vi "attribute_read_int32.vi"(5 "Repeated Capability":string, 7 "Attribute":T1={"Identifier"="", "Descriptive name"="", "Data Type"=enum."Integer 32", "Command"="", "Access"=2, "Range Table"="", "Read Callback"="", "Write Callback"="", "Range Callback"="", "Check Callback"="", "Rngtable Callback"="", "Coerce Callback"="", "Supported Models"="", "Instrument Options"="", "Repeated Capabilities"="", "Check Status Callback"="", "Index"=0, "Flag: OPC Wait"=FALSE, "Flag: Dont check status"=FALSE, "Flag: Cache Only"=FALSE} {"Access" items=["Read Only", "Write Only", "Read/Write"]}, 8 "error in":errorcluster, 11 "VISA resource name":refnum<visa-resource-name>) -> (0 "error out":errorcluster, 2 "I32 out":i32, 3 "VISA resource name out":refnum<visa-resource-name>)   [LabVIEW 2014, in "rszvl_rsidr_core.lvlib"]
uses:
  rszvl_rsidr_core.lvlib
  type_Attribute.ctl
  type_Attribute_Data_Type.ctl
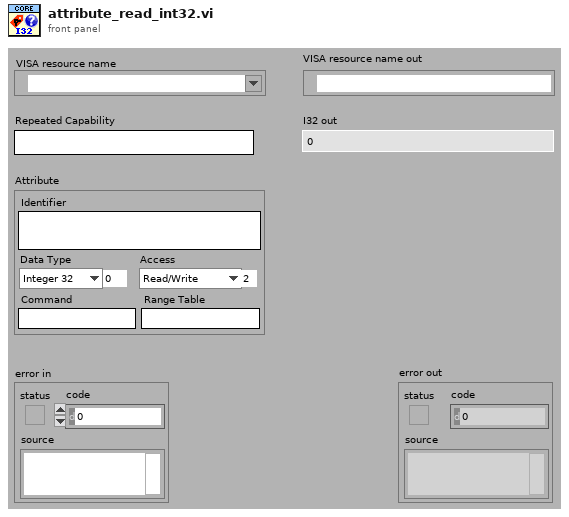
[diagram p1: front panel]
types:
  T1 = typedef "rszvl_rsidr_core.lvlib/type_Attribute.ctl" = cluster{"Identifier":string, "Descriptive name":string, "Data Type":T2, "Command":string, "Access":u16, "Range Table":string, "Read Callback":string, "Write Callback":string, "Range Callback":string, "Check Callback":string, "Rngtable Callback":string, "Coerce Callback":string, "Supported Models":string, "Instrument Options":string, "Repeated Capabilities":string, "Check Status Callback":string, "Index":i32, "Flag: OPC Wait":bool, "Flag: Dont check status":bool, "Flag: Cache Only":bool}
  T2 = typedef "rszvl_rsidr_core.lvlib/type_Attribute_Data_Type.ctl" = enum16{"Integer 32", "Double", "String", "Boolean", "None", "Integer 64"}
  T3 = typedef "rszvl_rsidr_core.lvlib/type_Session_Data.ctl" = cluster{"Instr type":string, "Instr type for err. msg.":string, "Installed Options":string[], "OPC Timeout":i32, "Query Instrument Status":bool, "Check Range":bool, "Check Options":bool, "Add LF to Write":bool, "Simulate":bool, "Logging":bool, "Logging params":variant, "Interface Type":enum16{"Unknown", "GPIB", "VXI", "GPIB_VXI", "ASRL", "PXI", "TCPIP", "USB", "SOCKET"}, "Fast Sweep":i32, "AdditionalFlags":i32, "WaitBeforeWrite":i32, "WaitBeforeRead":i32, "BinDataChunkSize":i64}
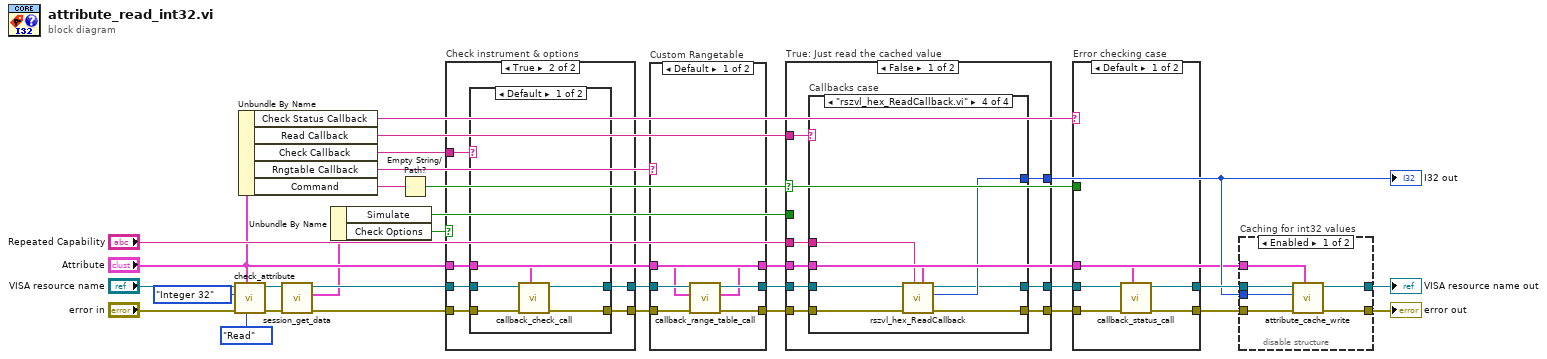
[diagram p0: block diagram]
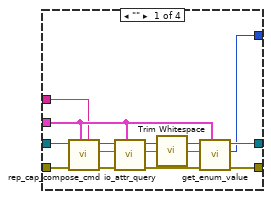
[diagram p2: hidden frame]
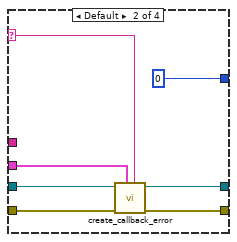
[diagram p3: hidden frame]
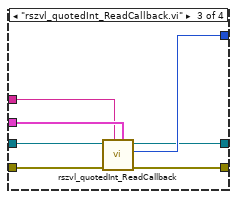
[diagram p4: hidden frame]
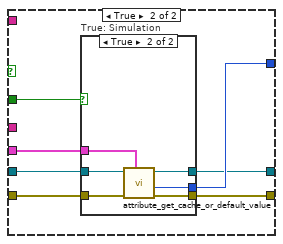
[diagram p5: hidden frame]
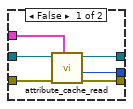
[diagram p6: hidden frame]
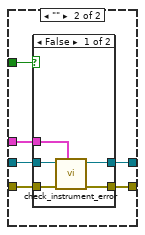
[diagram p8: hidden frame]
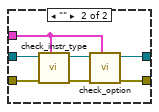
[diagram p11: hidden frame]
diagram:
  n1 = call "check_attribute.vi"("Access"=enum16{"Read", "Write"}."Read", "Attribute"="Attribute", "error in"="error in", "Data Type"=type_Attribute_Data_Type."Integer 32", "VISA resource name"="VISA resource name") -> ("error out"=w16:errorcluster, "VISA resource name out"=w17:refnum<visa-resource-name>)  [unwired: 5 in]
  n2 = Unbundle By Name("Attribute") -> ("Check Status Callback"=w18:string, "Read Callback"=w19:string, "Check Callback"=w7:string, "Rngtable Callback"=w8:string, "Command"=w3:string)
  n3 = call "session_get_data.vi"("error in"=w16, "VISA resource name"=w17) -> ("error out"=w15:errorcluster, "Session User Data out"=w2:T3, "VISA resource name out"=w14:refnum<visa-resource-name>)  [unwired: 7 in]
  n4 = Unbundle By Name(w2) -> ("Simulate"=w1:bool, "Check Options"=w13:bool)
  n5 = Empty String/Path?(string/path=w3) -> (empty?=w28:bool)
  n6 = case "Check instrument & options" shown="True" w13 {
    tunnel: [w33 w39] -> w12
    tunnel: [w32 w38] -> w11
    tunnel: w7 -> [_ w37]
    tunnel: w15 -> [w32 w36]
    tunnel: w14 -> [w33 w35]
    tunnel: "Attribute" -> [_ w34]
    frame False {
    }
    frame True {
      n7 = case shown="Default" w37 {
        tunnel: [w43 w49] -> w39
        tunnel: [w41 w48] -> w38
        tunnel: w36 -> [w42 w47]
        tunnel: w35 -> [w44 w46]
        tunnel: w34 -> [w40 w45]
        frame Default {
          n8 = call "callback_check_call.vi"("Attribute"=w40, "error in"=w42, "VISA resource name"=w44) -> ("error out"=w41:errorcluster, "VISA resource name out"=w43:refnum<visa-resource-name>)  [unwired: 7 in]
        }
        frame "" {
          n9 = call "check_instr_type.vi"("Attribute"=w45, "error in"=w47, "VISA resource name"=w46) -> ("error out"=w51:errorcluster, "VISA resource name out"=w50:refnum<visa-resource-name>)  [unwired: 6 in, 1 out]
          n10 = call "check_option.vi"("Attribute"=w45, "error in"=w51, "VISA resource name"=w50) -> ("error out"=w48:errorcluster, "VISA resource name out"=w49:refnum<visa-resource-name>)  [unwired: 7 in]
        }
      }
    }
  }
  n11 = case "Custom Rangetable" shown="Default" w8 {
    tunnel: w12 -> [w57 w60]
    tunnel: w11 -> [w54 w59]
    tunnel: [w56 w60] -> w10
    tunnel: [w55 w59] -> w9
    tunnel: "Attribute" -> [w53 w58]
    tunnel: [w52 w58] -> w6
    frame Default {
      n12 = call "callback_range_table_call.vi"("error in"=w54, "Attribute in"=w53, "VISA resource name"=w57) -> ("error out"=w55:errorcluster, "Attribute out"=w52:T1, "VISA resource name out"=w56:refnum<visa-resource-name>)  [unwired: 6 in]
    }
    frame "" {
    }
  }
  n13 = case "True: Just read the cached value" shown="False" w28 {
    tunnel: "Repeated Capability" -> [w68 _]
    tunnel: [w67 w106] -> w21
    tunnel: [w66 w105] -> w20
    tunnel: [w65 w107] -> w23
    tunnel: w19 -> [w64 _]
    tunnel: w10 -> [w63 w109]
    tunnel: w9 -> [w62 w110]
    tunnel: w6 -> [w61 w108]
    tunnel: w1 -> [_ w104]
    frame False {
      n14 = case "Callbacks case" shown="\"rszvl_hex_ReadCallback.vi\"" w64 {
        selector: w64 -> [_ w84 _ _]
        tunnel: w63 -> [w82 w88 w95 w102]
        tunnel: w62 -> [w81 w89 w96 w103]
        tunnel: w68 -> [w74 _ w93 w100]
        tunnel: [w80 w86 w90 w97] -> w66
        tunnel: [w79 w87 w91 w98] -> w67
        tunnel: [w69 0 ("Attribute Value I32") w92 w99] -> w65
        tunnel: w61 -> [w75 w85 w94 w101]
        frame "" {
          n15 = call "rep_cap_compose_cmd.vi"("Repeated Capability"=w74, "Attribute"=w75, "error in"=w81, "VISA resource name"=w82) -> ("error out"=w78:errorcluster, "Command out"=w77:string, "VISA resource name out"=w76:refnum<visa-resource-name>)  [unwired: 5 in]
          n16 = call "io_attr_query.vi"("Attribute"=w75, "error in"=w78, "write buffer"=w77, "VISA resource name"=w76) -> ("error out"=w73:errorcluster, "read buffer"=w71:string, "VISA resource name out"=w72:refnum<visa-resource-name>)  [unwired: 5 in]
          n17 = call "Trim Whitespace.vi"("string"=w71) -> ("trimmed string"=w70:string)  [unwired: 1 in]
          n18 = call "get_enum_value.vi"("Attribute"=w75, "error in"=w73, "String Value"=w70, "VISA resource name"=w72) -> ("error out"=w79:errorcluster, "I32 output"=w69:i32, "VISA resource name out"=w80:refnum<visa-resource-name>)  [unwired: 5 in]
        }
        frame Default {
          n19 = call "create_callback_error.vi"("Callback Name"=w84, "Attribute"=w85, "error in"=w89, "VISA resource name"=w88) -> ("error out"=w87:errorcluster, "VISA resource name out"=w86:refnum<visa-resource-name>)  [unwired: 6 in]
        }
        frame "rszvl_quotedInt_ReadCallback.vi" {
          n20 = call "rszvl_quotedInt_ReadCallback.vi"("Attribute"=w94, "Repeated Capability"=w93, "error in"=w96, "VISA resource name"=w95) -> ("error out"=w91:errorcluster, "Attribute Value I32"=w92:i32, "VISA resource name out"=w90:refnum<visa-resource-name>)  [unwired: 5 in]
        }
        frame "rszvl_hex_ReadCallback.vi" {
          n21 = call "rszvl_hex_ReadCallback.vi"("Attribute"=w101, "Repeated Capability"=w100, "error in"=w103, "VISA resource name"=w102) -> ("error out"=w98:errorcluster, "Attribute Value I32"=w99:i32, "VISA resource name out"=w97:refnum<visa-resource-name>)  [unwired: 5 in]
        }
      }
    }
    frame True {
      n22 = case "True: Simulation" shown="True" w104 {
        tunnel: w110 -> [w116 w122]
        tunnel: w109 -> [w115 w121]
        tunnel: w108 -> [w114 w117]
        tunnel: [w113 w118] -> w107
        tunnel: [w112 w120] -> w106
        tunnel: [w111 w119] -> w105
        frame False {
          n23 = call "attribute_cache_read.vi"("Attribute"=w114, "error in"=w116, "VISA resource name"=w115) -> ("error out"=w112:errorcluster, "Integer 32 out"=w113:i32, "VISA resource name out"=w111:refnum<visa-resource-name>)  [unwired: 1 in, 5 out]
        }
        frame True {
          n24 = call "attribute_get_cache_or_default_value.vi"("Attribute"=w117, "error in"=w122, "VISA resource name"=w121) -> ("error out"=w120:errorcluster, "Integer 32 out"=w118:i32, "VISA resource name out"=w119:refnum<visa-resource-name>)  [unwired: 1 in, 5 out]
        }
      }
    }
  }
  "I32 out" <- w23
  n25 = case "Error checking case" shown="Default" w18 {
    tunnel: w21 -> [w127 w131]
    tunnel: [w126 w130] -> w27
    tunnel: [w125 w132] -> w26
    tunnel: w20 -> [w124 w133]
    tunnel: w6 -> [w123 w129]
    tunnel: w28 -> [_ w128]
    frame Default {
      n26 = call "callback_status_call.vi"("Attribute"=w123, "error in"=w127, "VISA resource name"=w124) -> ("error out"=w126:errorcluster, "VISA resource name out"=w125:refnum<visa-resource-name>)  [unwired: 7 in]
    }
    frame "" {
      n27 = case shown="False" w128 {
        tunnel: w133 -> [w138 w140]
        tunnel: [w137 w140] -> w132
        tunnel: w131 -> [w136 w139]
        tunnel: [w135 w139] -> w130
        tunnel: w129 -> [w134 _]
        frame False {
          n28 = call "check_instrument_error.vi"("Attribute"=w134, "error in"=w136, "VISA resource name"=w138) -> ("error out"=w135:errorcluster, "VISA resource name out"=w137:refnum<visa-resource-name>)  [unwired: 7 in]
        }
        frame True {
        }
      }
    }
  }
  n29 = disable-structure "Caching for int32 values" shown="Enabled" {
    disable-tunnel: [w146 w148] -> w25
    disable-tunnel: [w145 w147] -> w24
    disable-tunnel: w27 -> [w144 w147]
    disable-tunnel: w26 -> [w143 w148]
    disable-tunnel: w23 -> [w142 _]
    disable-tunnel: "Attribute" -> [w141 _]
    frame Enabled {
      n30 = call "attribute_cache_write.vi"("Attribute"=w141, "error in"=w144, "Value in"=w142, "VISA resource name"=w143) -> ("error out"=w145:errorcluster, "VISA resource name out"=w146:refnum<visa-resource-name>)  [unwired: 6 in]
    }
    frame Disabled {
    }
  }
  "error out" <- w24
  "VISA resource name out" <- w25
